vi "fgv_agv_cmd-val.vi"(7 "cmd":T2=enum."init stop", 9 "limits in":T1={"limit_linear-v"=0.0, "limit_angular-v"=0.2}, 11 "agv_speed_in":cluster{"v_linear":dbl, "v_angular":dbl}={"v_linear"=0.5, "v_angular"=0.0}) -> (1 "limits out":T1={"limit_linear-v"=0.0, "limit_angular-v"=0.2}, 3 "agv_speed_out":cluster{"v_linear":dbl, "v_angular":dbl})   [LabVIEW 2019]
uses:
  Ctrl/agv_cmd_v.ctl
  Ctrl/obstacle_info.ctl
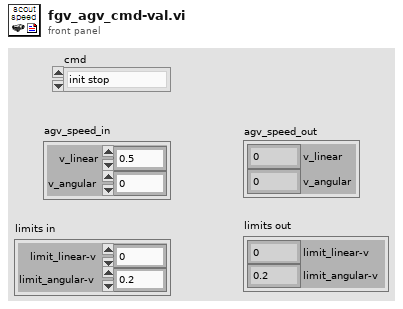
[diagram p1: front panel]
types:
  T1 = cluster{"limit_linear-v":dbl, "limit_angular-v":dbl}
  T2 = typedef "agv_cmd_v.ctl" = enum16{"write limit", "init stop", "write", "read"}
  T3 = typedef "obstacle_info.ctl" = enum16{"init", "read", "obstacle status in", "write limit", "inrange pt-n"}
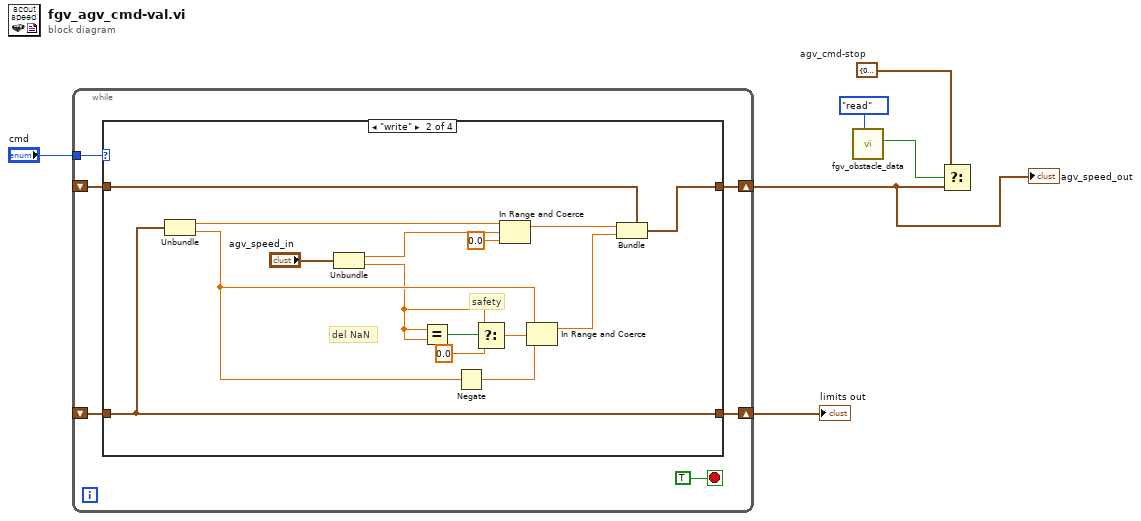
[diagram p0: block diagram]
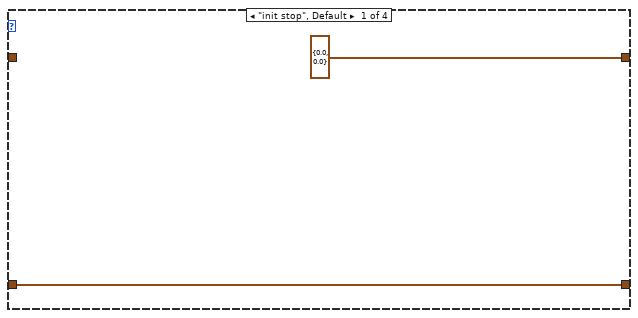
[diagram p2: hidden frame]
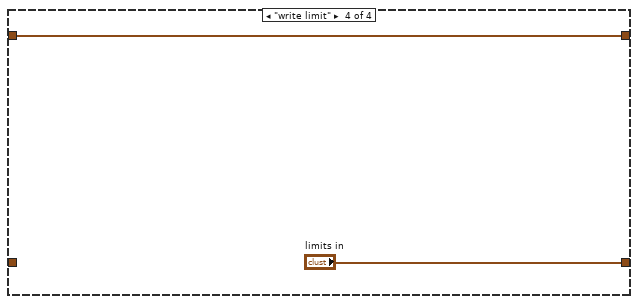
[diagram p4: hidden frame]
diagram:
  w3 = cluster{"v_linear":dbl, "v_angular":dbl} {"v_linear"=0.0, "v_angular"=0.0}  # agv_cmd-stop
  n1 = while {
    tunnel: "cmd" -> [w11]
    shift-right: [w10] -> w1
    shift-left: _ -> [w9]
    shift-right: [w8] -> w2
    shift-left: _ -> [w7]
    stop <- TRUE stop-if-true
    n2 = case shown="\"write\"" w11 {
      tunnel: [cluster{"v_linear":dbl, "v_angular":dbl} {"v_linear"=0.0, "v_angular"=0.0} ("agv_cmd") w16 w31 w32] -> w10
      tunnel: w9 -> [_ w18 w31 w32]
      tunnel: [w13 w25 w30 "limits in"] -> w8
      tunnel: w7 -> [w13 w25 w30 _]
      frame "init stop", Default {
      }
      frame "write" {
        # "del NaN"
        # "safety"
        n3 = Unbundle(w25) -> ("limit_linear-v"=w15:dbl, "limit_angular-v"=w24:dbl)
        n4 = Unbundle("agv_speed_in") -> ("v_linear"=w21:dbl, "v_angular"=w20:dbl)
        n5 = Equal?(x=w20, y=w20) -> (x = y?=w28:bool)
        n6 = Negate(x=w24) -> (-x=w29:dbl)
        n7 = Select(t=w20, s=w28, f=0.0) -> (s? t:f=w27:dbl)
        n8 = In Range and Coerce(upper limit=w15, x=w21, lower limit=0.0 ("하위 리미트")) -> (coerced(x)=w19:dbl)  [unwired: 1 out]
        n9 = In Range and Coerce(upper limit=w24, x=w27, lower limit=w29) -> (coerced(x)=w17:dbl)  [unwired: 1 out]
        n10 = Bundle(cluster=w18, "v_linear"=w19, "v_angular"=w17) -> (w16:cluster{"v_linear":dbl, "v_angular":dbl})
      }
      frame "read" {
      }
      frame "write limit" {
      }
    }
  }
  "agv_speed_out" <- w1
  "limits out" <- w2
  n11 = call "fgv_obstacle_data.vi"("cmd"=obstacle_info."read") -> ("obstacle out"=w4:bool)  [unwired: 7 in, 3 out]
  n12 = Select(t=w3, s=w4, f=w1) -> ()  [unwired: 1 out]
